vi "2D_zeros.vi"(10 "column_number":i32, 11 "row_number":i32) -> (3 "2D_Rand":dbl[][](array[numeric]))   [LabVIEW 2014]
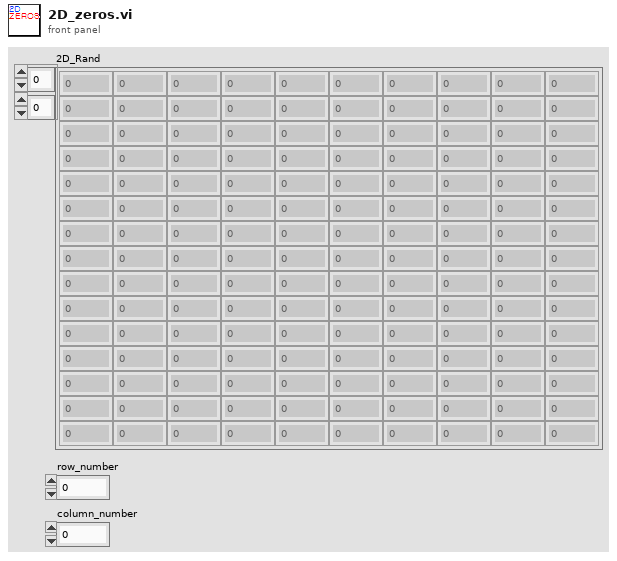
[diagram p1: front panel]
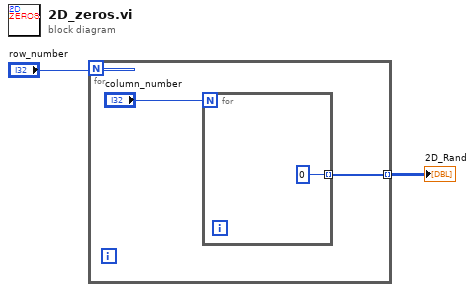
[diagram p0: block diagram]
diagram:
  n1 = for {
    N: "row_number" -> [_]
    tunnel: [w4] -> w2 mode=indexing
    n2 = for {
      N: "column_number" -> [_]
      tunnel: [0] -> w4 mode=indexing
    }
  }
  "2D_Rand" <- w2
